vi "Load lvlibp path.vi"(7 "Class Name":string, 8 "error in":errorcluster, 11 "Configuration in":refnum<class "Configuration.lvclass">) -> (0 "error out":errorcluster, 2 "lvlibp Path":path, 3 "Configuration out":refnum<class "Configuration.lvclass">)   [LabVIEW 2018, in "Configuration.lvlib" / "Configuration.lvclass"]
doc: "This program will load the path to a packed project library.\n\nIt is contingent on a packed project library being built. If a packed project library is not found, it will return a <Not A Path> filepath and an error -43."
uses:
  Configuration.lvclass
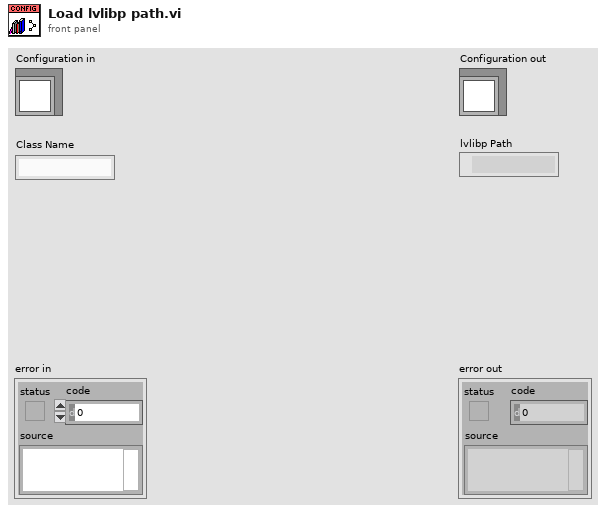
[diagram p1: front panel]
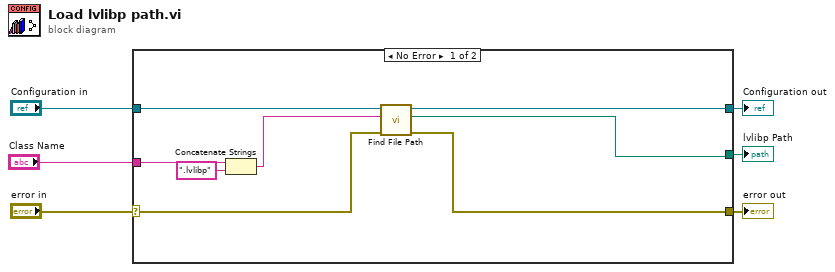
[diagram p0: block diagram]
diagram:
  n1 = case shown="No Error" "error in" {
    selector: "error in" -> [w10 w16]
    tunnel: [w9 w16] -> w5
    tunnel: [w11 w15] -> w3
    tunnel: "Configuration in" -> [w12 w15]
    tunnel: "Class Name" -> [w14 _]
    tunnel: [w8 _] -> w1
    frame No Error {
      n2 = Concatenate Strings(w14, ".lvlibp" ("string")) -> (w7:string)
      n3 = call "Find File Path.vi"("error in"=w10, "Filename"=w7, "Configuration in"=w12) -> ("error out"=w9:errorcluster, "File Path"=w8:path, "Configuration out"=w11:refnum<class "Configuration.lvclass">)  [unwired: 6 in]
    }
    frame Error {
    }
  }
  "error out" <- w5
  "Configuration out" <- w3
  "lvlibp Path" <- w1
